vi "Get IConfigure.vi"(8 "Error In":errorcluster, 11 "reference in":refnum<class "Thermometer Multichannel.lvclass">) -> (0 "Error Out":errorcluster, 2 "IConfigure":refnum<class "IConfigure.lvclass">, 3 "reference out":refnum<class "Thermometer Multichannel.lvclass">)   [LabVIEW 2024, in "Thermometer Multichannel.lvclass"]
uses:
  Thermometer Multichannel.lvclass
  Interfaces/IConfigure/IConfigure.lvclass
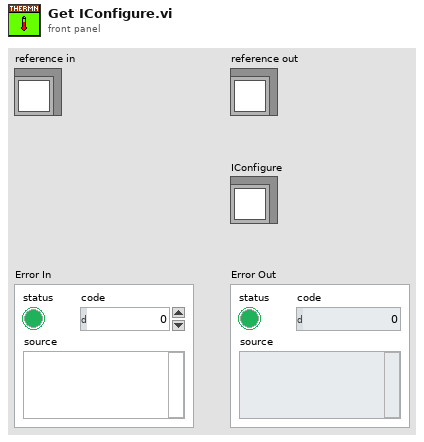
[diagram p1: front panel]
types:
  T1 = typedef "Thermometer Multichannel.lvclass/ObjectAttributes.ctl" = cluster{"IConfigure":refnum<class "IConfigure.lvclass">, "Worker Enqueuer":refnum<class "Message Enqueuer.lvclass">}
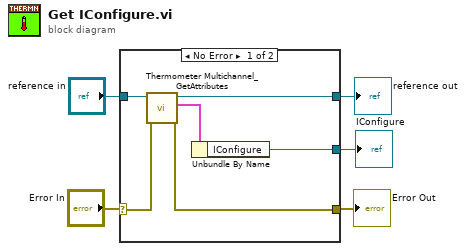
[diagram p0: block diagram]
diagram:
  n1 = case shown="No Error" "Error In" {
    selector: "Error In" -> [w11 w13]
    tunnel: [w9 w13] -> w4
    tunnel: [w7 w12] -> w2
    tunnel: "reference in" -> [w8 w12]
    tunnel: [w6 _] -> w1
    frame No Error {
      n2 = call "Thermometer Multichannel_GetAttributes.vi"("Error In"=w11, "reference in"=w8) -> ("Error Out"=w9:errorcluster, "Data"=w10:T1, "reference out"=w7:refnum<class "Thermometer Multichannel.lvclass">)  [unwired: 6 in, 1 out]
      n3 = Unbundle By Name(w10) -> ("IConfigure"=w6:refnum<class "IConfigure.lvclass">)
    }
    frame Error {
    }
  }
  "Error Out" <- w4
  "reference out" <- w2
  "IConfigure" <- w1
